vi "用户管理.vi"(9 "权限":i32, 10 "用户名":string, 11 "用户信息":string[][](array[string])) -> (3 "项名":string[][](array[string]))   [LabVIEW 2020]
uses:
  <vilib>/Utility/miscctls.llb/LVRowAndColumnTypeDef.ctl
  <vilib>/Utility/file.llb/Write Delimited Spreadsheet (string).vi
panel:
  out "项名 2":string[][](array[string])
  out "单元格位置":T1
  out "子数组":string[][](array[string])
  in  "Btn_Exit":bool
  in  "Btn_Modify":bool
  in  "Btn_Del":bool
  in  "Btn_Add":bool
  in  "多列列表框":i32(listbox)
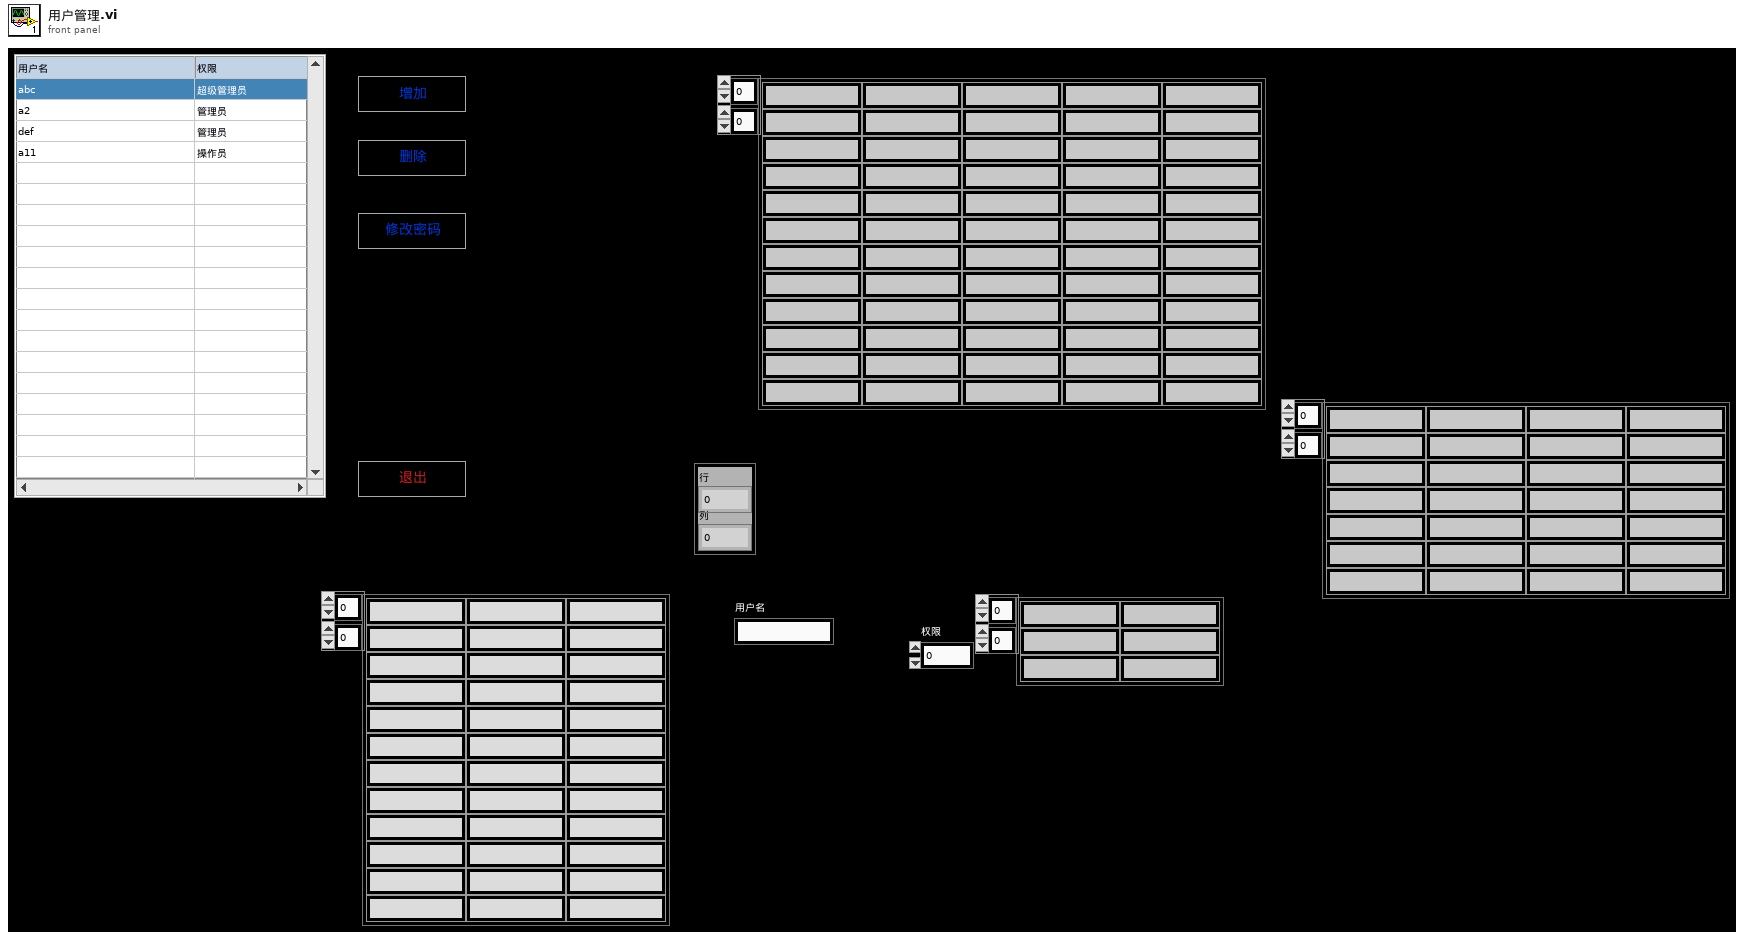
[diagram p1: front panel]
types:
  T1 = typedef "LVRowAndColumnTypeDef.ctl" = cluster{"Row":i32, "Column":i32}
  T2 = typedef "LVPoint32TypeDef.ctl" = cluster{"Horizontal":i32, "Vertical":i32}
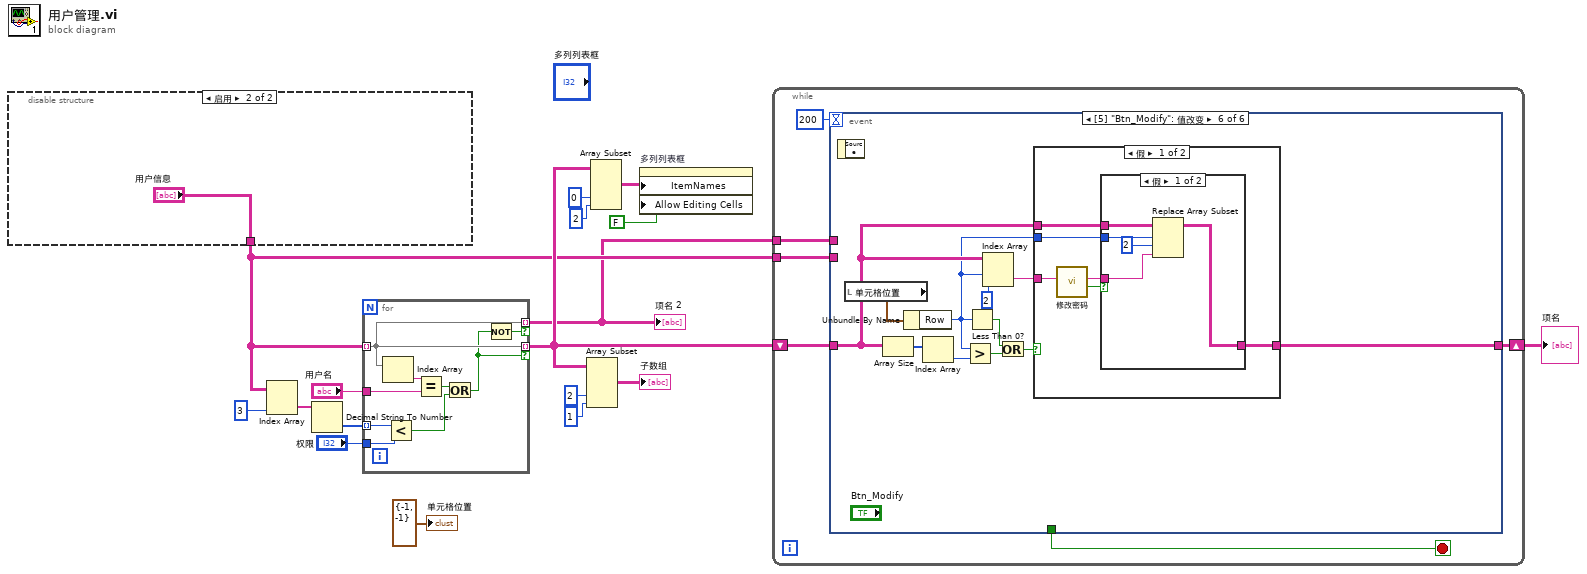
[diagram p0: block diagram]
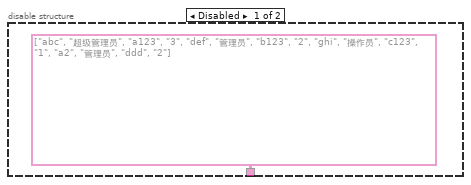
[diagram p2: hidden frame]
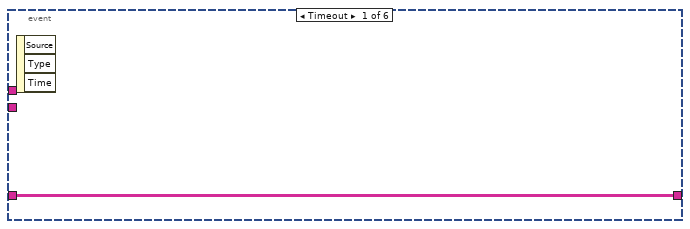
[diagram p3: hidden frame]
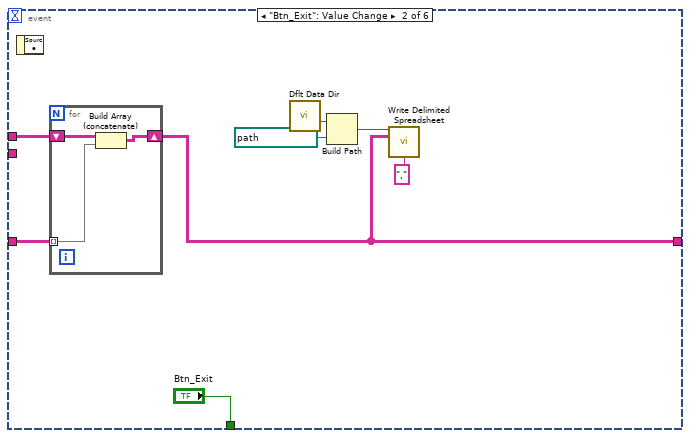
[diagram p4: hidden frame]
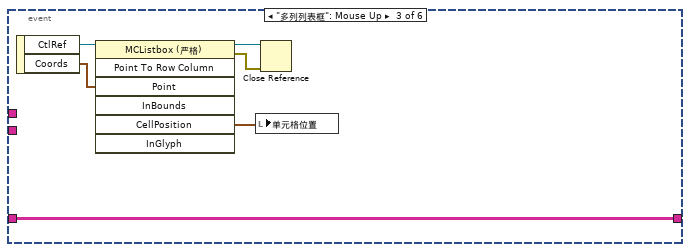
[diagram p5: hidden frame]
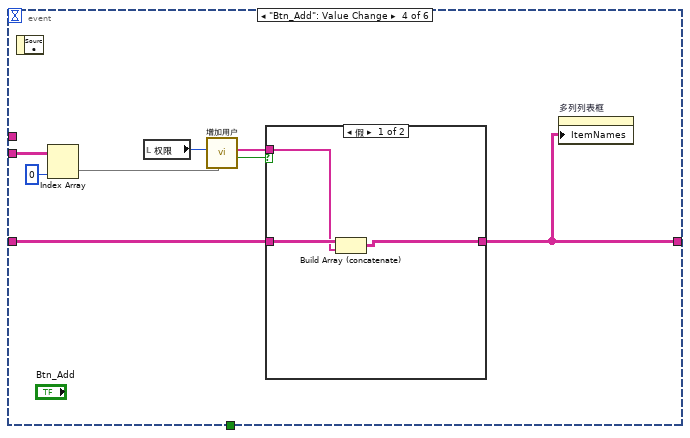
[diagram p6: hidden frame]
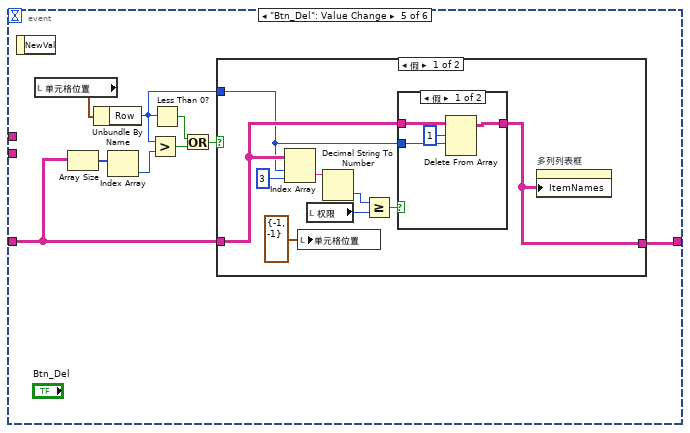
[diagram p8: hidden frame]
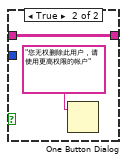
[diagram p9: hidden frame]
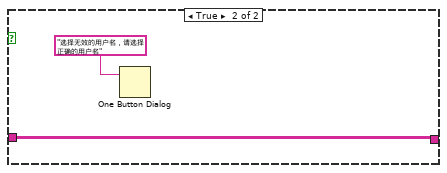
[diagram p10: hidden frame]
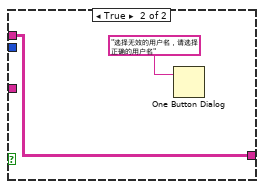
[diagram p12: hidden frame]
diagram:
  n1 = disable-structure shown="启用" {
    disable-tunnel: [string[][] [["abc", "超级管理员", "a123", "3"], ["def", "管理员", "b123", "2"], ["ghi", "操作员", "c123", "1"], ["a2", "管理员", "ddd", "2"]] ("项名") "用户信息"] -> w6
    frame Disabled {
    }
    frame Enabled {
    }
  }
  n2 = Index Array(array=w6, index (col)=3 ("索引")) -> (element=w10:string[])  [unwired: 1 in]
  n3 = Decimal String To Number(string=w10) -> (number=w9:i32[])  [unwired: 2 in, 1 out]
  n4 = for {
    tunnel: w6 -> [w22] mode=indexing
    tunnel: "权限" -> [w27]
    tunnel: w9 -> [w28] mode=indexing
    tunnel: [w22] -> w7 mode=indexing if=w21
    tunnel: "用户名" -> [w25]
    tunnel: [w22] -> w1 mode=indexing if=w20
    n5 = Index Array(array=w22) -> (element=w26:string)  [unwired: 1 in]
    n6 = Less?(x=w28, y=w27) -> (x < y?=w23:bool)
    n7 = Equal?(x=w26, y=w25) -> (x = y?=w24:bool)
    n8 = Or(x=w24, y=w23) -> (x .or. y?=w21:bool)
    n9 = Not(x=w21) -> (.not. x?=w20:bool)
  }
  "项名 2" <- w1
  n10 = Array Subset(array=w7, index (col)=2 ("索引"), length (col)=1 ("索引")) -> (→"子数组":string[][])  [unwired: 2 in]
  n11 = Array Subset(array=w7, index (col)=0 ("索引"), length (col)=2 ("索引")) -> (w8:string[][])  [unwired: 2 in]
  n12 = property on="多列列表框" class="MCListbox (严格)"("ItemNames"=w8, "Allow Editing Cells"=FALSE ("允许编辑单元格")) -> ()  [unwired: 2 in, 2 out]
  n13 = while {
    shift-right: [w30] -> w5
    shift-left: w7 -> [w32]
    tunnel: w6 -> [w31]
    tunnel: w1 -> [w29]
    stop <- w33 stop-if-true
    n14 = event shown="[5] \"Btn_Modify\": 值改变" {
      selector: _ -> [_ _ _ _ _ _]
      dyn-events: _ -> [_ _ _ _ _ _]
      timeout: 200 -> [_ _ _ _ _ _]
      tunnel: [_ "Btn_Exit" _ _ _ _] -> w33
      tunnel: w32 -> [w35 w42 w48 w58 w68 w93]
      tunnel: w31 -> [_ _ _ w56 _ _]
      tunnel: [w35 w37 w48 w53 w67 w92] -> w30
      tunnel: w29 -> [_ w41 _ _ _ _]
      event Timeout {
        n15 = event-data() -> ()  [unwired: 1 in, 3 out]
      }
      event "Btn_Exit": Value Change {
        n16 = event-data() -> ()  [unwired: 1 in, 1 out]
        n17 = for {
          shift-right: [w44] -> w37
          shift-left: w41 -> [w46]
          tunnel: w42 -> [w45] mode=indexing
          n18 = Build Array (concatenate)(w46, w45) -> (w44:string[][])
        }
        n19 = call <vilib>:"Dflt Data Dir.vi"() -> ("App:Default Data Directory"=w40:path)
        n20 = Build Path(base path=w40, name or relative path=path "用户管理.csv" ("名称或相对路径")) -> (appended path=w38:path)
        n21 = call-poly <vilib>:"Write Delimited Spreadsheet.vi"("file path (dialog if empty)"=w38, "2D data"=w37, "delimiter (\\t)"="," ("delimiter (\\t)")) -> ()  [unwired: 11 in, 2 out]
      }
      event "多列列表框": Mouse Up {
        n22 = event-data() -> ("CtlRef"=w52:refnum<vi>, "Coords"=w51:T2)  [unwired: 1 in]
        n23 = invoke class="MCListbox (严格)" method="Point To Row Column"(reference=w52, "Point"=w51) -> (reference out=w50:refnum<vi>, error out=w49:errorcluster, "CellPosition"=w47:T1)  [unwired: 5 in, 4 out]
        n24 = local write "单元格位置"(w47) -> ()
        n25 = Close Reference(reference=w50, error in (no error)=w49) -> ()  [unwired: 1 out]
      }
      event "Btn_Add": Value Change {
        n26 = event-data() -> ()  [unwired: 1 in, 1 out]
        n27 = Index Array(array=w56, index (col)=0 ("禁用的索引 (列)")) -> (element=w54:string[])  [unwired: 1 in]
        n28 = local read "权限"() -> (w60:i32)
        n29 = call "增加用户.vi"("用户名in"=w54, "权限in"=w60) -> ("取消"=w59:bool, "用户信息"=w57:string[])  [unwired: 8 in]
        n30 = case shown="假" w59 {
          tunnel: w58 -> [w63 w64]
          tunnel: [w61 w64] -> w53
          tunnel: w57 -> [w62 _]
          frame False {
            n31 = Build Array (concatenate)(w63, w62) -> (w61:string[][])
          }
          frame True {
          }
        }
        n32 = property on="多列列表框" class="MCListbox (严格)"("ItemNames"=w53) -> ()  [unwired: 2 in, 2 out]
      }
      event "Btn_Del": Value Change {
        n33 = event-data() -> ()  [unwired: 1 in, 1 out]
        n34 = local read "单元格位置"() -> (w66:T1)
        n35 = Array Size(array=w68) -> (size(s)=w73:i32[])
        n36 = Unbundle By Name(w66) -> ("Row"=w65:i32)
        n37 = Index Array(array=w73) -> (element=w72:i32)  [unwired: 1 in]
        n38 = Greater?(x=w65, y=w72) -> (0:w70:bool)
        n39 = Less Than 0?(x=w65) -> (x < 0?=w71:bool)
        n40 = Or(x=w71, y=w70) -> (x .or. y?=w69:bool)
        n41 = case shown="假" w69 {
          tunnel: w68 -> [w80 w89]
          tunnel: [w81 w89] -> w67
          tunnel: w65 -> [w79 _]
          frame False {
            n42 = Index Array(array=w80, index (row)=w79, index (col)=3 ("禁用的索引 (列)")) -> (element=w77:string)
            n43 = local write "单元格位置"(T1 {"Row"=-1, "Column"=-1} ("单元格位置")) -> ()
            n44 = local read "权限"() -> (w75:i32)
            n45 = Decimal String To Number(string=w77) -> (number=w76:i32)  [unwired: 2 in, 1 out]
            n46 = Greater Or Equal?(x=w76, y=w75) -> (x >= y?=w74:bool)
            n47 = case shown="假" w74 {
              tunnel: [w85 w87] -> w81
              tunnel: w80 -> [w84 w87]
              tunnel: w79 -> [w83 _]
              frame False {
                n48 = Delete From Array(array=w84, length=1 ("长度"), index (row)=w83) -> (array with subset deleted=w85:string[][])  [unwired: 1 in, 1 out]
              }
              frame True {
                n49 = One Button Dialog(message="您无权删除此用户，请使用更高权限的帐户" ("消息")) -> ()  [unwired: 1 in, 1 out]
              }
            }
            n50 = property on="多列列表框" class="MCListbox (严格)"("ItemNames"=w81) -> ()  [unwired: 2 in, 2 out]
          }
          frame True {
            n51 = One Button Dialog(message="选择无效的用户名，请选择正确的用户名" ("消息")) -> ()  [unwired: 1 in, 1 out]
          }
        }
      }
      event "Btn_Modify": Value Change {
        n52 = event-data() -> ()  [unwired: 1 in, 1 out]
        n53 = local read "单元格位置"() -> (w97:T1)
        n54 = Array Size(array=w93) -> (size(s)=w101:i32[])
        n55 = Unbundle By Name(w97) -> ("Row"=w91:i32)
        n56 = Index Array(array=w101) -> (element=w100:i32)  [unwired: 1 in]
        n57 = Greater?(x=w91, y=w100) -> (0:w98:bool)
        n58 = Less Than 0?(x=w91) -> (x < 0?=w99:bool)
        n59 = Index Array(array=w93, index (row)=w91, index (col)=2 ("禁用的索引 (列)")) -> (element=w94:string)
        n60 = Or(x=w99, y=w98) -> (x .or. y?=w96:bool)
        n61 = case shown="假" w96 {
          tunnel: w94 -> [w107 _]
          tunnel: w93 -> [w106 w115]
          tunnel: [w102 w115] -> w92
          tunnel: w91 -> [w104 _]
          frame False {
            n62 = call "修改密码.vi"("旧密码in"=w107) -> ("取消"=w105:bool, "新密码out"=w103:string)  [unwired: 9 in]
            n63 = case shown="假" w105 {
              tunnel: w106 -> [w112 w113]
              tunnel: w104 -> [w111 _]
              tunnel: w103 -> [w109 _]
              tunnel: [w108 w113] -> w102
              frame False {
                n64 = Replace Array Subset(array=w112, new element=w109, index (row)=w111, index (col)=2 ("禁用的索引 (列)")) -> (w108:string[][])
              }
              frame True {
              }
            }
          }
          frame True {
            n65 = One Button Dialog(message="选择无效的用户名，请选择正确的用户名" ("消息")) -> ()  [unwired: 1 in, 1 out]
          }
        }
      }
    }
  }
  "项名" <- w5
  "单元格位置" <- T1 {"Row"=-1, "Column"=-1} ("单元格位置")
